vi "Read Temperature Measured.vi"(11 "TemperatureSensor in":refnum<class "TemperatureSensor.lvclass">) -> (2 "Temperature Measured":dbl[unit]=274.15 min=274.15 max=573.15 format="%.1f", 3 "TemperatureSensor out":refnum<class "TemperatureSensor.lvclass">)   [LabVIEW 2013, in "TemperatureSensor.lvclass"]
uses:
  TemperatureSensor.lvclass
  TemperatureSensor.lvclass/TemperatureSensor.ctl
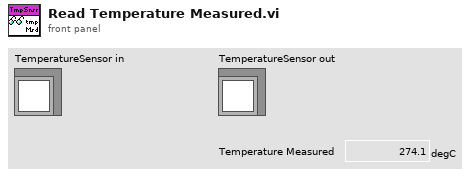
[diagram p1: front panel]
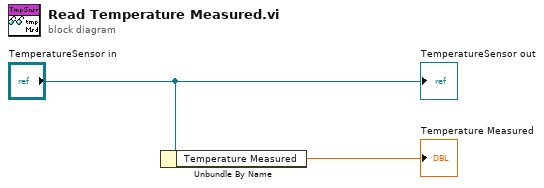
[diagram p0: block diagram]
diagram:
  n1 = Unbundle By Name("TemperatureSensor in") -> ("Temperature Measured"=→"Temperature Measured":dbl[unit])
  "TemperatureSensor out" <- "TemperatureSensor in"
